vi "Leggi filtro ed etichette.vi"(10 "ID COLLEGAMENTO":i32, 11 "LINGUA":i32) -> (0 "INDEX COPPIA":i32, 1 "INDICI":i32[](array[numeric]), 2 "FILTRO":bool[](array[boolean]), 3 "ETICHETTE":string[](array[string]), 4 "INDEX CORRENTE":i32, 5 "ALL":string[](array[string]))   [LabVIEW 2019]
uses:
  <vilib>/Utility/file.llb/Read Delimited Spreadsheet (string).vi
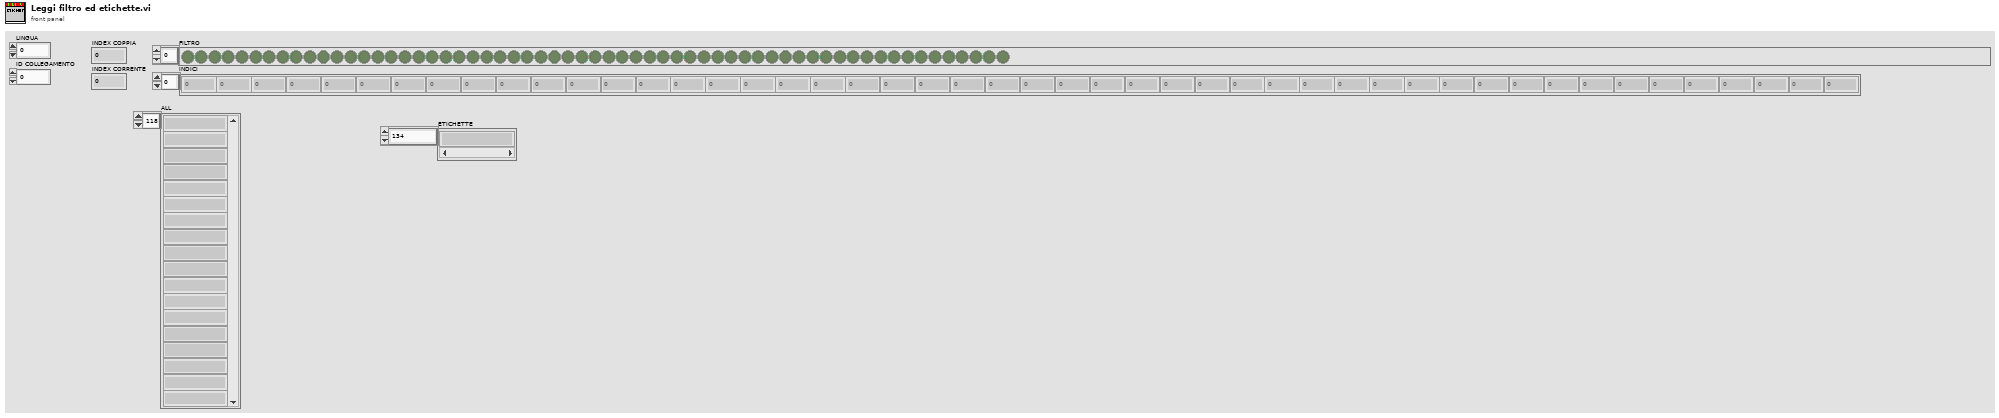
[diagram p1: front panel]
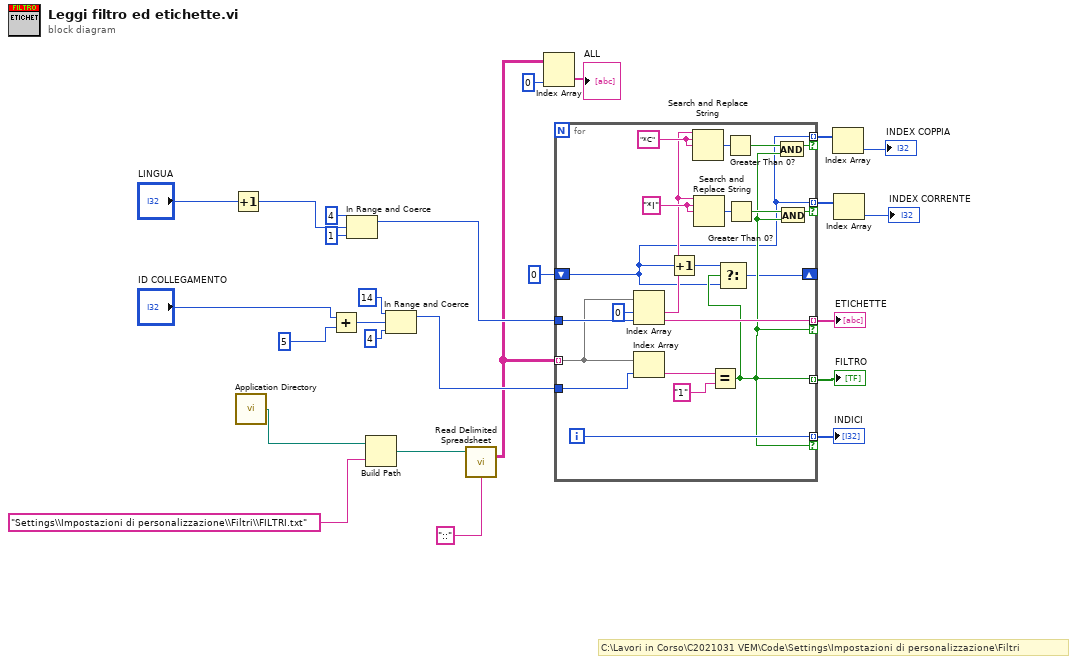
[diagram p0: block diagram]
diagram:
  # "C:\\Lavori in Corso\\C2021031 VEM\\Code\\Settings\\Impostazioni di personalizzazione\\Filtri"
  n1 = Increment(x="LINGUA") -> (x+1=w10:i32)
  n2 = call <vilib>:"Application Directory.vi"() -> ("Application Directory"=w1:path)
  n3 = Add(x="ID COLLEGAMENTO", y=5) -> (x+y=w15:i32)
  n4 = In Range and Coerce(upper limit=4, x=w10, lower limit=1) -> (coerced(x)=w16:i32)  [unwired: 1 out]
  n5 = Build Path(base path=w1, name or relative path="Settings\\Impostazioni di personalizzazione\\Filtri\\FILTRI.txt") -> (appended path=w25:path)
  n6 = In Range and Coerce(upper limit=14, x=w15, lower limit=4) -> (coerced(x)=w14:i32)  [unwired: 1 out]
  n7 = call-poly <vilib>:"Read Delimited Spreadsheet.vi"("file path (dialog if empty)"=w25, "delimiter (\\t)"="::" ("delimiter (\\t)")) -> ("all rows"=w2:string[][])  [unwired: 8 in, 5 out]
  n8 = Index Array(array=w2, index (col)=0 ("disabled index (col)")) -> (element=→"ALL":string[])  [unwired: 1 in]
  n9 = for {
    tunnel: w2 -> [w42] mode=indexing
    tunnel: w16 -> [w47]
    tunnel: [w46] -> w21 mode=indexing if=w30
    tunnel: w14 -> [w45]
    tunnel: [w30] -> w20 mode=indexing
    tunnel: [w34] -> w11 mode=indexing if=w30
    tunnel: [w27] -> w9 mode=indexing if=w33
    tunnel: [w27] -> w8 mode=indexing if=w31
    shift-right: [w28] -> _
    shift-left: 0 -> [w27]
    i -> [w34]
    w36 = "*I" ("search string")
    w40 = "*C" ("search string")
    n10 = Index Array(array=w42, index #1=0 ("index"), index #2=w47) -> (element #1=w35:string, element #2=w46:string)
    n11 = Index Array(array=w42, index=w45) -> (element=w44:string)
    n12 = Increment(x=w27) -> (x+1=w29:i32)
    n13 = Search and Replace String(input string=w35, search string=w40, replace string=w40) -> (number of replacements=w39:i32)  [unwired: 5 in, 3 out]
    n14 = Search and Replace String(input string=w35, search string=w36, replace string=w36) -> (number of replacements=w37:i32)  [unwired: 5 in, 3 out]
    n15 = Equal?(x=w44, y="1") -> (x = y?=w30:bool)
    n16 = Select(t=w29, s=w30, f=w27) -> (s? t:f=w28:i32)
    n17 = Greater Than 0?(x=w39) -> (x > 0?=w38:bool)
    n18 = Greater Than 0?(x=w37) -> (x > 0?=w32:bool)
    n19 = And(x=w38, y=w30) -> (x .and. y?=w33:bool)
    n20 = And(x=w32, y=w30) -> (x .and. y?=w31:bool)
  }
  "ETICHETTE" <- w21
  "FILTRO" <- w20
  "INDICI" <- w11
  n21 = Index Array(array=w9) -> (element=→"INDEX COPPIA":i32)  [unwired: 1 in]
  n22 = Index Array(array=w8) -> (element=→"INDEX CORRENTE":i32)  [unwired: 1 in]
